vi "dfd_Group Delay_Generate Ideal Response and Weight.vi"(7 "p":dbl, 8 "weight for grid":dbl[](array[numeric]), 10 "fgrid":dbl[](array[numeric]), 11 "band specification":T1[](array[typedef]) {"subband specs"."weight" format="%.2f"}) -> (0 "weight":dbl[](array[numeric]), 1 "desired response":dbl[](array[numeric]), 2 "fgrid (dup)":dbl[](array[numeric]), 3 "band specification (dup)":T1[](array[typedef]) {"subband specs"."weight" format="%.2f"})   [LabVIEW 2017, in "NI_DigFilter_Design.lvlib"]
uses:
  <vilib>/addons/Digital Filter Design/NI_DigFilter_Design.lvlib
  <vilib>/addons/Digital Filter Design/_GroupDelay.llb/dfd_Group Delay_Band Spec.ctl
  <vilib>/addons/Digital Filter Design/NI_DigFilterLicensed.lvlib
panel:
  # "freq"
  # "group delay"
  # "weight"
  # "freq"
  # "group delay"
  # "weight"
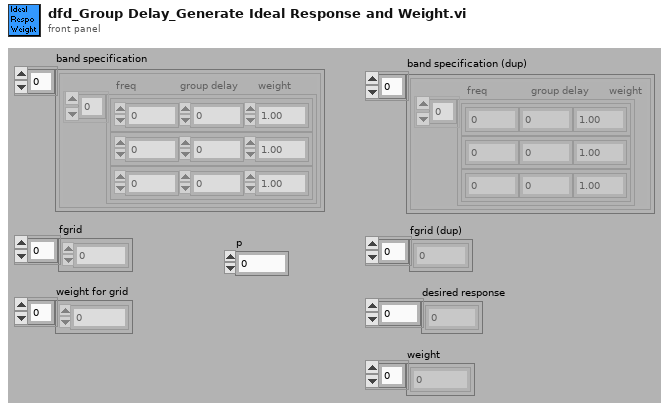
[diagram p1: front panel]
types:
  T1 = typedef "NI_DigFilterLicensed.lvlib/dfd_Group Delay_Band Spec.ctl" = cluster{"subband specs":cluster{"freq":dbl, "group delay":dbl, "weight":dbl}[]}
  T2 = cluster{"freq":dbl, "group delay":dbl, "weight":dbl}[]
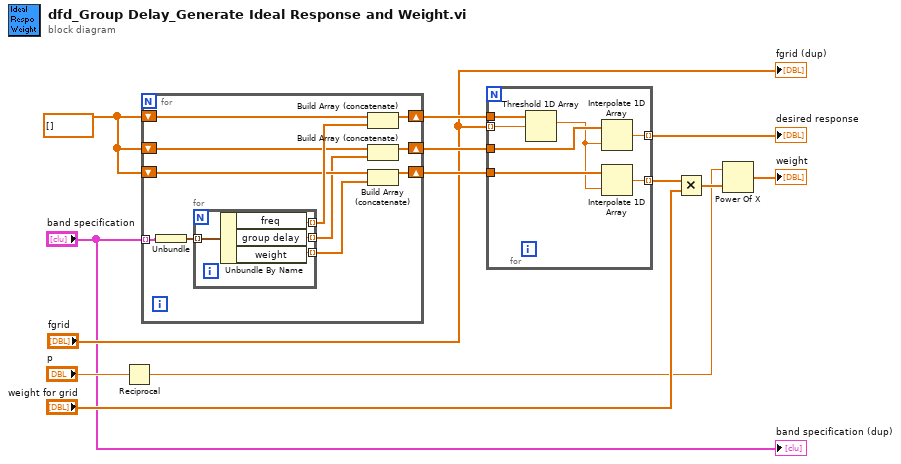
[diagram p0: block diagram]
diagram:
  w13 = dbl[] []
  n1 = Reciprocal(x="p") -> (1/x=w3:dbl)
  n2 = for {
    tunnel: "band specification" -> [w16] mode=indexing
    shift-right: [w24] -> w12
    shift-left: w13 -> [w22]
    shift-right: [w21] -> w11
    shift-left: w13 -> [w20]
    shift-right: [w18] -> w10
    shift-left: w13 -> [w19]
    n3 = Unbundle(w16) -> ("subband specs"=w15:T2)
    n4 = for {
      tunnel: w15 -> [w28] mode=indexing
      tunnel: [w27] -> w17 mode=indexing
      tunnel: [w26] -> w23 mode=indexing
      tunnel: [w25] -> w14 mode=indexing
      n5 = Unbundle By Name(w28) -> ("freq"=w26:dbl, "group delay"=w27:dbl, "weight"=w25:dbl)
    }
    n6 = Build Array (concatenate)(w22, w23) -> (w24:dbl[])
    n7 = Build Array (concatenate)(w20, w17) -> (w21:dbl[])
    n8 = Build Array (concatenate)(w19, w14) -> (w18:dbl[])
  }
  n9 = for {
    tunnel: "fgrid" -> [w34] mode=indexing
    tunnel: w12 -> [w35]
    tunnel: w11 -> [w33]
    tunnel: [w32] -> w7 mode=indexing
    tunnel: w10 -> [w31]
    tunnel: [w29] -> w9 mode=indexing
    n10 = Threshold 1D Array(2:w34, 3:w35) -> (0:w30:dbl)  [unwired: 1 out]
    n11 = Interpolate 1D Array(1:w30, 2:w33) -> (0:w32:dbl)
    n12 = Interpolate 1D Array(1:w30, 2:w31) -> (0:w29:dbl)
  }
  "desired response" <- w7
  n13 = Multiply(x=w9, y="weight for grid") -> (x*y=w5:dbl[])
  n14 = Power Of X(1:w5, 2:w3) -> (0:→"weight":dbl[])
  "fgrid (dup)" <- "fgrid"
  "band specification (dup)" <- "band specification"
